vi "UpdateMasterCluster.vi"(6 "MainQ":refnum<queue>, 8 "ErrorIn":errorcluster, 11 "HWClusterIn":T1={"FPGA"={"Target"=enum."1", "Channel"=enum."4", "Ref1"=refnum, "Ref2"=refnum}}) -> (0 "ErrorOut":errorcluster, 3 "HWClusterOut":T1={"FPGA"={"Target"=enum."1", "Channel"=enum."4", "Ref1"=refnum, "Ref2"=refnum}})   [LabVIEW 2018]
doc: "Adds the MasterCluster (<B>ClusterIn</B>) into the queue member \"Q\" of the MasterCluster and sets the next state of the Main (Consumer) Loop to RfrshPnl (RefreshPanel). \n\nThis also updates the functional global with the latest MasterCluster.\n\n<B>ClusterOut</B> is the updated version of <B>ClusterIn</B> with the new queue element and next state.\n\nProducer loops, such as the Hardware Loop should call this whenever they have updated state information and need to feed this up to the Main (Consumer) Loop.\n\nCopyright © 2011 Epimedia, Inc. All Rights Reserved.\n\nThe Epimedia Application Library is Copyright © 2009-2011 Epimedia, Inc. \nAll Rights Reserved. Used under license."
uses:
  Controls/HWCluster.ctl
  Controls/Clusts/FPGA_Config_Clust.ctl
  Controls/Enums/TargetNumber.ctl
  Queue/RTMainQueueElements.ctl
panel:
  # "Copyright © 2011 Epimedia, Inc. All Rights Reserved.\n\nThe Epimedia Application Library is Copyright © 2009-2011 Epimedia, Inc. \nAll Rights Reserved. Used under license."
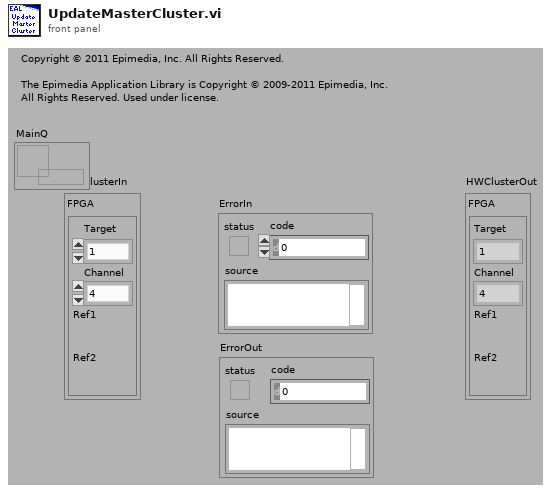
[diagram p1: front panel]
types:
  T1 = typedef "HWCluster.ctl" = cluster{"FPGA":T2}
  T2 = typedef "FPGA_Config_Clust.ctl" = cluster{"Target":T3, "Channel":T3, "Ref1":refnum<k20>, "Ref2":refnum<k20>}
  T3 = typedef "TargetNumber.ctl" = enum16{"1", "2", "3", "4"}
  T4 = typedef "RTMainQueueElements.ctl" = enum16{"RTMain_InitQ", "RTMain_InitSW", "RTMain_InitCtrls", "RTMain_ReInitHW", "RTMain_FromStream", "RTMain_StrtHWLp", "RTMain_UpdtHWClstr", "RTMain_Start", "RTMain_Stop", "RTMain_Error", "RTMain_Config", "RTMain_Exit"}
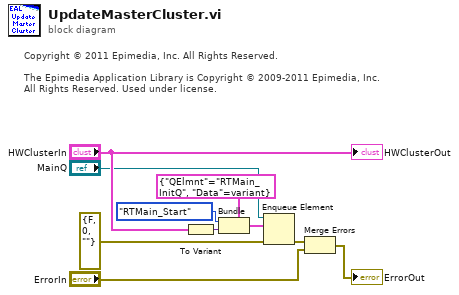
[diagram p0: block diagram]
diagram:
  # "Copyright © 2011 Epimedia, Inc. All Rights Reserved.\n\nThe Epimedia Application Library is Copyright © 2009-2011 Epimedia, Inc. \nAll Rights Reserved. Used under license."
  n1 = To Variant(anything="HWClusterIn") -> (Variant=w8:variant)
  n2 = Bundle(cluster=cluster{"QElmnt":T4, "Data":variant} {"QElmnt"=enum."RTMain_InitQ", "Data"=variant} ("Cluster"), "QElmnt"=RTMainQueueElements."RTMain_Start", "Data"=w8) -> (w7:cluster{"QElmnt":T4, "Data":variant})
  n3 = Enqueue Element(queue="MainQ", element=w7, error in (no error)=errorcluster {"status"=FALSE, "code"=0, "source"=""}) -> (error out=w3:errorcluster)  [unwired: 3 out]
  n4 = Merge Errors(w3, "ErrorIn") -> (→"ErrorOut":errorcluster)
  "HWClusterOut" <- "HWClusterIn"
